vi "OP400ZP_prep bdd iso.vi"(8 "tabin":string[](array[string]), 10 "InsuP":string, 11 "InsuN":string) -> (0 "tabout":string[](array[string]))   [LabVIEW 2020]
uses:
  OP400ZP_selectdata.ctl
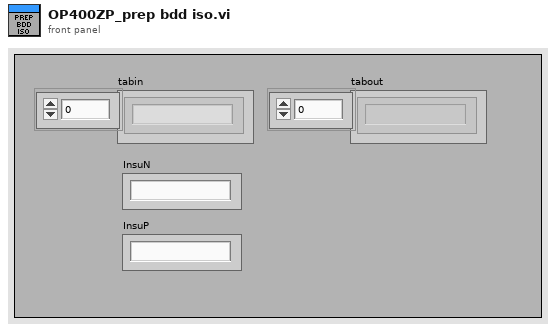
[diagram p1: front panel]
types:
  T1 = typedef "OP400ZP_selectdata.ctl" = u16
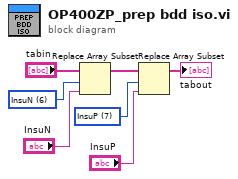
[diagram p0: block diagram]
diagram:
  w1 = T1 7 items=["IdOp300", "DateStart", "DeltaTC", "DeltaVC", "ImageVers", "IniFileVers", "InsuN", "InsuP", "MCU", "OCV", "Operateur", "Pass", "SN", "SoftVers", "TC0", "TC1", "TempsTest", "Tfactory", "Type", "VC0", "VC1"] ("Menu déroulant")
  w2 = T1 6 items=["IdOp300", "DateStart", "DeltaTC", "DeltaVC", "ImageVers", "IniFileVers", "InsuN", "InsuP", "MCU", "OCV", "Operateur", "Pass", "SN", "SoftVers", "TC0", "TC1", "TempsTest", "Tfactory", "Type", "VC0", "VC1"] ("Menu déroulant")
  n1 = Replace Array Subset(array="tabin", new element="InsuN", index=w2) -> (w5:string[])
  n2 = Replace Array Subset(array=w5, new element="InsuP", index=w1) -> (→"tabout":string[])
